vi "Clamp Wrapper.vi"(0 "Limit Max":bool, 1 "In":bool, 2 "Beam Breaker":bool, 3 "Limit Min":bool, 4 "Out":bool) -> ()   [LabVIEW 2014]
uses:
  Precreated VIs/Robot Global Data.vi
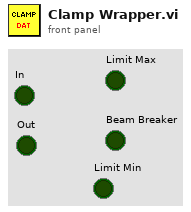
[diagram p1: front panel]
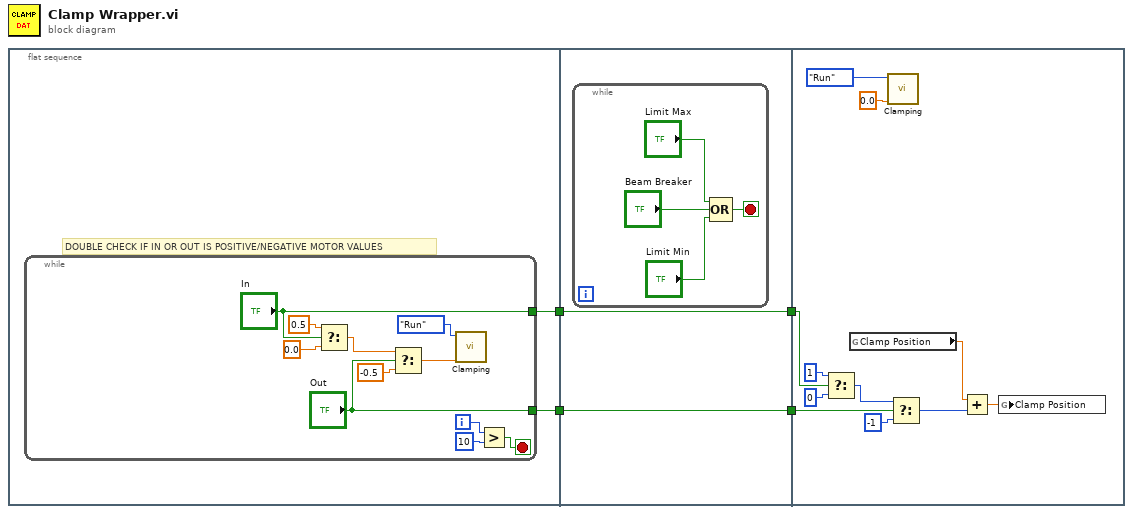
[diagram p0: block diagram]
diagram:
  n1 = flat-sequence {
    tunnel: [w6] -> w3
    tunnel: [w5] -> w1
    tunnel: [w19] -> w4
    tunnel: w3 -> [w19]
    tunnel: [w18] -> w2
    tunnel: w1 -> [w18]
    tunnel: w4 -> [w30]
    tunnel: w2 -> [w24]
    frame #0 {
      # "DOUBLE CHECK IF IN OR OUT IS POSITIVE/NEGATIVE MOTOR VALUES"
      n2 = while {
        tunnel: ["In"] -> w6
        tunnel: ["Out"] -> w5
        i -> [w15]
        stop <- w13 stop-if-true
        n3 = Select(t=0.5, s="In", f=0.0) -> (s? t:f=w10:dbl)
        n4 = Select(t=w10, s="Out", f=-0.5) -> (s? t:f=w11:dbl)
        n5 = call "Clamping.vi"("Motor Speed"=w11, "Mode"=enum8{"Start", "Run", "Finish"}."Run") -> ()  [unwired: 10 in]
        n6 = Greater?(x=w15, y=10) -> (0:w13:bool)
      }
    }
    frame #1 {
      n7 = while {
        stop <- w23 stop-if-true
        n8 = Compound Arithmetic op=OR("Limit Max", "Beam Breaker", "Limit Min") -> (w23:bool)
      }
    }
    frame #2 {
      n9 = Select(t=1, s=w30, f=0) -> (s? t:f=w25:i32)
      n10 = global read "Robot Global Data.vi" "Clamp Position"() -> (w32:dbl)
      n11 = call "Clamping.vi"("Motor Speed"=0.0, "Mode"=enum8{"Start", "Run", "Finish"}."Run") -> ()  [unwired: 10 in]
      n12 = Select(t=w25, s=w24, f=-1) -> (s? t:f=w26:i32)
      n13 = Add(x=w32, y=w26) -> (x+y=w31:dbl)
      n14 = global write "Robot Global Data.vi" "Clamp Position"(w31) -> ()
    }
  }
